vi "TestVision1.vi"(7 "error in":errorcluster) -> (27 "error out":errorcluster)   [LabVIEW 2020]
uses:
  <vilib>/vision/NI_Vision_Development_Module.lvlib
panel:
  out "Image Out":T1(plugin-control)
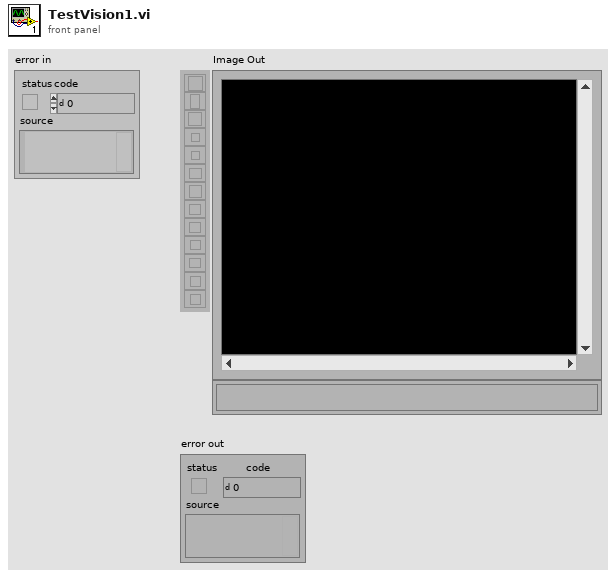
[diagram p1: front panel]
types:
  T1 = typedef "IMAQ Image.ctl" = refnum<image>
  T2 = cluster{"Measurement Parameter":i32, "Range Lower Value":dbl, "Range Upper Value":dbl, "Range":bool, "Measurement Type":bool}[]
  T3 = cluster{"Brightness":sgl, "Contrast":sgl, "Gamma":sgl}
  T4 = typedef "Image Type" = u32
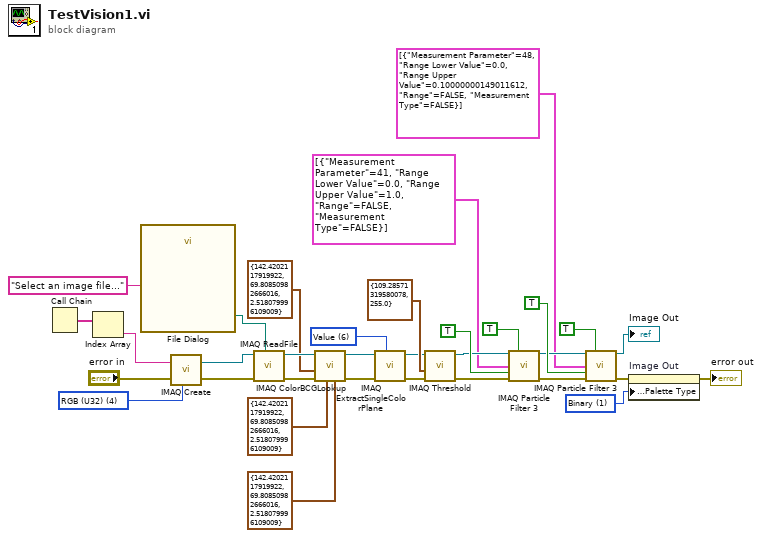
[diagram p0: block diagram]
diagram:
  w1 = u32 1 items=["Grayscale", "Binary", "Gradient", "Rainbow", "Temperature", "User Defined", "Binary 16 Bit", "Gradient 16 Bit", "Rainbow 16 Bit", "Temperature 16 Bit", "User Defined 16 Bit"] ("Palette Type")
  w20 = 6 items=["Red", "Green", "Blue", "Hue", "Saturation", "Luminance", "Value", "Intensity"] ("Color Plane")
  w26 = T4 4 items=["Grayscale (U8)", "Grayscale (I16)", "Grayscale (SGL)", "Complex (CSG)", "RGB (U32)", "HSL (U32)", "RGB (U64)", "Grayscale (U16)"] ("Image Type")
  n1 = Call Chain() -> (call chain=w30:string[])
  n2 = Index Array(array=w30) -> (element=w29:string)  [unwired: 1 in]
  n3 = call "File Dialog"("prompt"="Select an image file...") -> ("selected path"=w27:path)  [unwired: 6 in, 8 out]
  n4 = call "IMAQ Create"("Image Name"=w29, "Image Type"=w26, "error in (no error)"="error in") -> ("New Image"=w33:T1, "error out"=w32:errorcluster)  [unwired: 1 in, 1 out]
  n5 = call "IMAQ ReadFile"("File Path"=w27, "error in (no error)"=w32, "Image"=w33) -> ("error out"=w24:errorcluster, "Image Out"=w25:T1)  [unwired: 2 in, 5 out]
  n6 = call "IMAQ ColorBCGLookup"("Blue BCG Values"=T3 {"Brightness"=142.42021, "Contrast"=69.80851, "Gamma"=2.51808}, "Green BCG Values"=T3 {"Brightness"=142.42021, "Contrast"=69.80851, "Gamma"=2.51808}, "error in (no error)"=w24, "Red BCG Values"=T3 {"Brightness"=142.42021, "Contrast"=69.80851, "Gamma"=2.51808}, "Image Src"=w25) -> ("error out"=w18:errorcluster, "Image Dst Out"=w19:T1)  [unwired: 2 in, 3 out]
  n7 = call "IMAQ ExtractSingleColorPlane"("Color Plane"=w20, "error in (no error)"=w18, "Image Src"=w19) -> ("error out"=w15:errorcluster, "Image Dst Out"=w16:T1)  [unwired: 1 in, 6 out]
  n8 = call "IMAQ Threshold"("error in (no error)"=w15, "Range"=cluster{"Lower value":sgl, "Upper value":sgl} {"Lower value"=109.28571, "Upper value"=255.0}, "Image Src"=w16) -> ("error out"=w11:errorcluster, "Image Dst Out"=w12:T1)  [unwired: 3 in, 4 out]
  n9 = call "IMAQ Particle Filter 3"("Image Src"=w12, "Connectivity 4/8 (8)"=TRUE, "Selection Values"=T2 [{"Measurement Parameter"=41, "Range Lower Value"=0.0, "Range Upper Value"=1.0, "Range"=FALSE, "Measurement Type"=FALSE}], "Keep/Remove Particles (F)"=TRUE ("Keep/Remove Particles"), "error in (no error)"=w11) -> ("Image Dst Out"=w7:T1, "error out"=w6:errorcluster)  [unwired: 4 in, 5 out]
  n10 = call "IMAQ Particle Filter 3"("Image Src"=w7, "Connectivity 4/8 (8)"=TRUE, "Selection Values"=T2 [{"Measurement Parameter"=48, "Range Lower Value"=0.0, "Range Upper Value"=0.10000000149011612, "Range"=FALSE, "Measurement Type"=FALSE}], "Keep/Remove Particles (F)"=TRUE ("Keep/Remove Particles"), "error in (no error)"=w6) -> ("Image Dst Out"=→"Image Out":T1, "error out"=w4:errorcluster)  [unwired: 4 in, 5 out]
  n11 = property on="Image Out" class="ImageControl"(error in=w4, "Palette:Palette Type"=w1) -> (error out=→"error out":errorcluster)  [unwired: 1 in, 1 out]
